vi "Capture Example.vi"() -> ()   [LabVIEW 2020]
uses:
  g_ar_toolkit.image/CreateEmptyImageARGB.vi
  g_ar_toolkit.image/DrawImageToPictureARGB.vi
  g_ar_toolkit.image/CreateEmptyImageARGB.vi/3321fa97-f432-4e1e-8db9-a0df79aed21b.vi
  g_ar_toolkit.image/DrawImageToPictureARGB.vi/8cd07b1b-062e-4fe4-9e87-2eb3dc89fe0e.vi
  g_ar_toolkit.image/ARGBColourToU32.vi
  <vilib>/Utility/error.llb/Error Cluster From Error Code.vi
  g_ar_toolkit.capture/CameraStream/CameraStream.lvclass
  g_ar_toolkit.capture/CameraManager/CameraManager.lvclass
  g_ar_toolkit.image/g_ar_toolkit.image.lvlib
panel:
  in  "Start/Stop":bool
  in  "Format":string(combo)
  in  "Source":string(combo)
  in  "Enumerate":bool
  in  "Erase":bool
  in  "Picture Zoom":dbl=1.0 min=0.0001 max=10.0 step=0.1
  out "2D Picture":picture
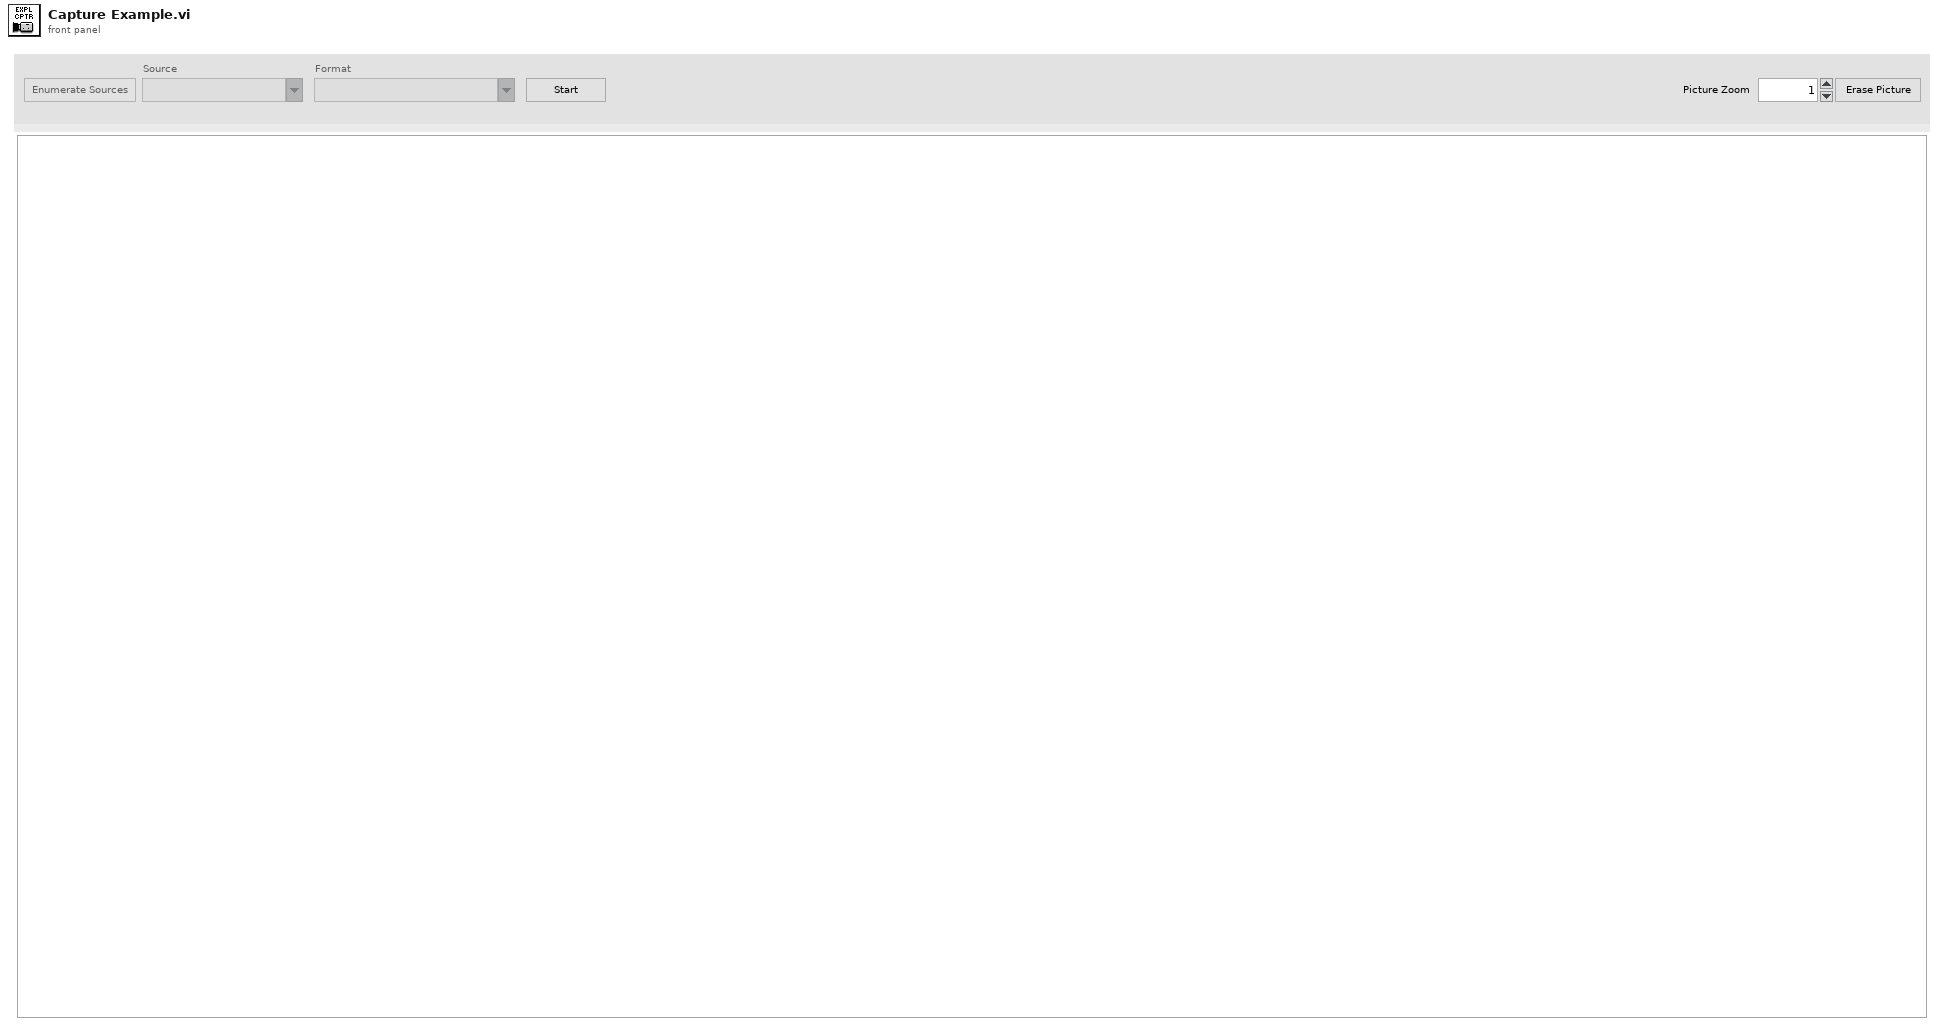
[diagram p1: front panel]
types:
  T1 = enum8{"Enabled", "Disabled", "Disabled and Grayed Out"}
  T2 = typedef "g_ar_toolkit.capture.lvlib/CameraManager.lvclass/Device Enumeration.ctl" = cluster{"Name":string, "Streams":set{cluster{"Parameters":T3, "Pixel-Format":u32, "Pixel-Format Name":string}}}
  T3 = typedef "g_ar_toolkit.capture.lvlib/CameraManager.lvclass/Stream Parameters.ctl" = cluster{"Width":u16, "Height":u16, "FPS":u8}
  T4 = set{cluster{"Parameters":T3, "Pixel-Format":u32, "Pixel-Format Name":string}}
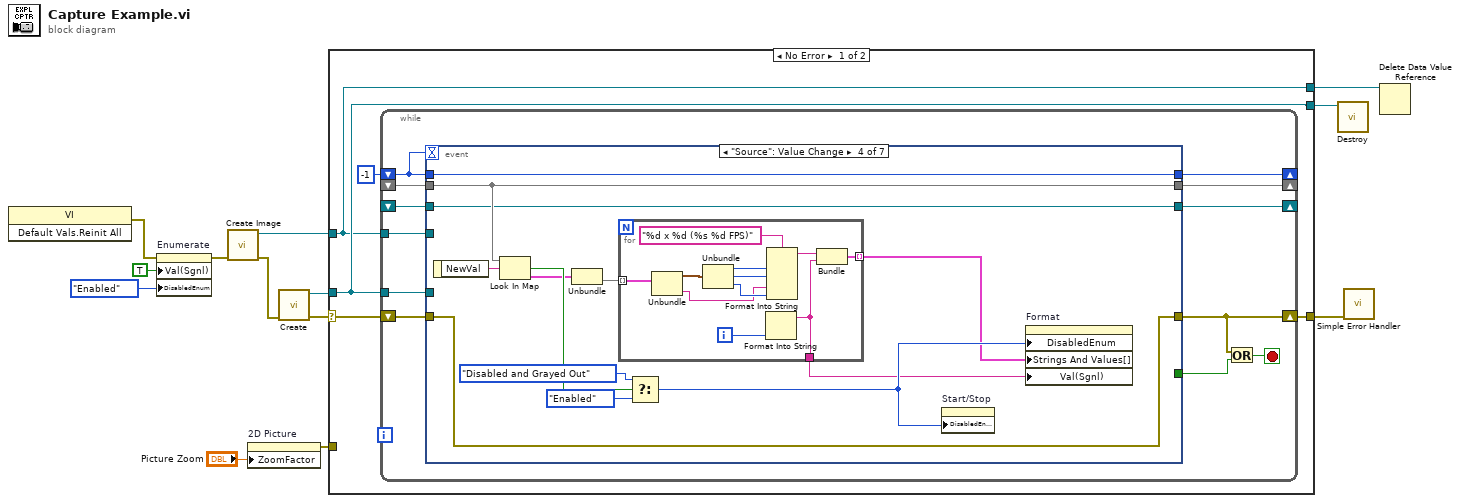
[diagram p0: block diagram]
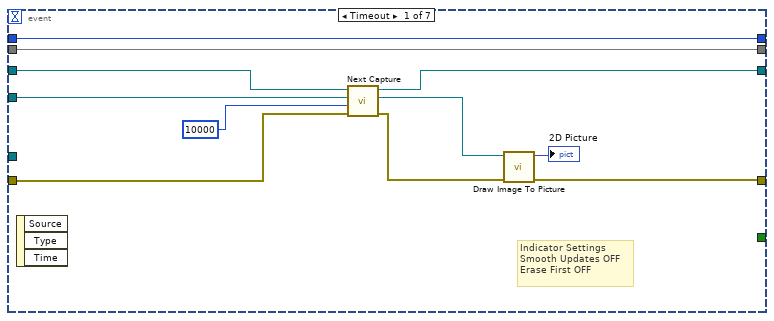
[diagram p2: hidden frame]
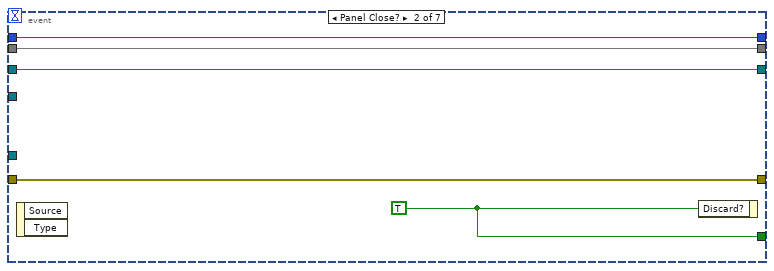
[diagram p3: hidden frame]
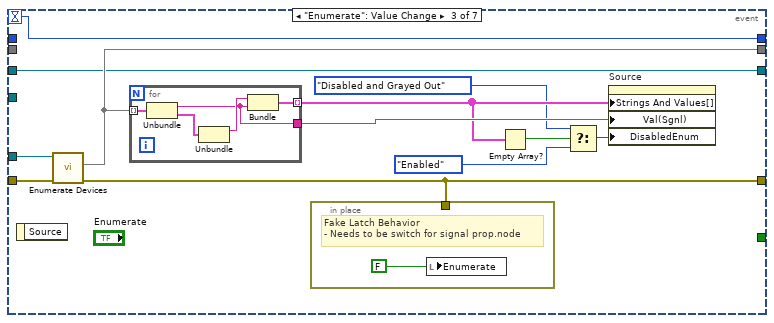
[diagram p4: hidden frame]
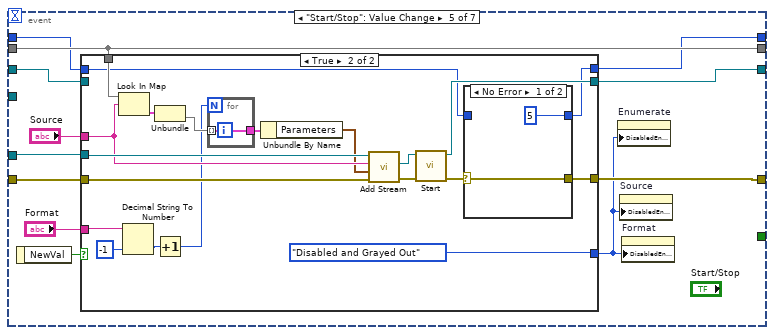
[diagram p5: hidden frame]
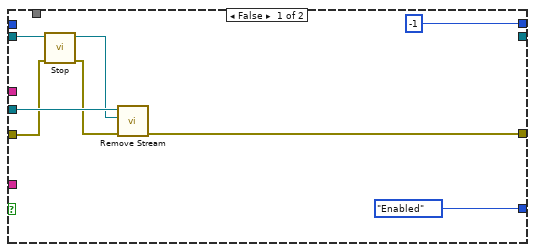
[diagram p6: hidden frame]
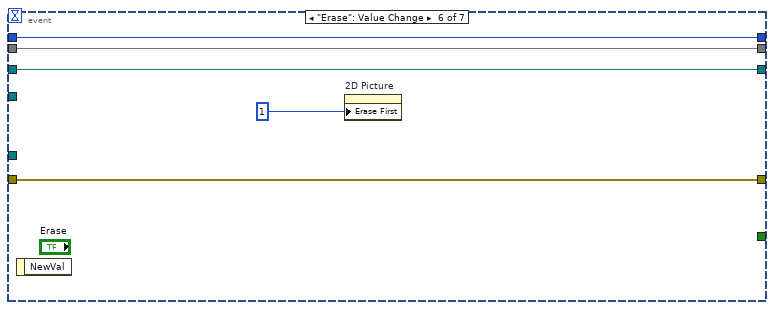
[diagram p8: hidden frame]
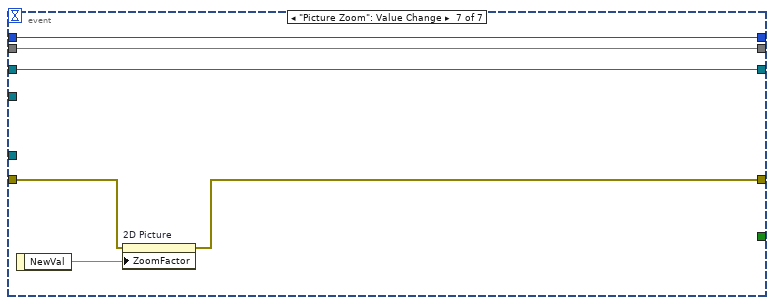
[diagram p9: hidden frame]
diagram:
  n1 = invoke class="VI" method="Default Vals.Reinit All"() -> (error out=w5:errorcluster)  [unwired: 3 in, 2 out]
  n2 = property on="Enumerate" class="Bool (strict)"(error in=w5, "Val(Sgnl)"=TRUE ("Value (Signaling)"), "DisabledEnum"=T1."Enabled" ("Disabled")) -> (error out=w1:errorcluster)  [unwired: 1 in, 1 out]
  n3 = call-poly "Create Image.vi"("error in (no error)"=w1) -> ("error out"=w4:errorcluster, "New ARGB Image"=w10:refnum<data-value>)  [unwired: 9 in]
  n4 = property on="2D Picture" class="Pict"("ZoomFactor"="Picture Zoom") -> (error out=w9:errorcluster)  [unwired: 2 in, 1 out]
  n5 = call "Create.vi"("error in (no error)"=w4) -> ("error out"=w13:errorcluster, "CameraManager"=w2:refnum<data-value>)  [unwired: 9 in]
  n6 = case shown="No Error" w13 {
    selector: w13 -> [w18 w145]
    tunnel: w2 -> [w17 w147]
    tunnel: [w17 w147] -> w12
    tunnel: w10 -> [w15 w146]
    tunnel: w9 -> [_ _]
    tunnel: [w15 w146] -> w7
    tunnel: [w14 w145] -> w6
    frame No Error {
      n7 = while {
        tunnel: w17 -> [w30]
        shift-right: [w28] -> _
        shift-left: _ -> [w27]
        shift-right: [w26] -> w14
        shift-left: w18 -> [w29]
        shift-right: [w23] -> _
        shift-left: -1 -> [w22]
        shift-right: [w21] -> _
        shift-left: _ -> [w20]
        tunnel: w15 -> [w19]
        stop <- w25 stop-if-true
        n8 = event shown="[3] \"Source\": Value Change" {
          selector: _ -> [_ _ _ _ _ _ _]
          dyn-events: _ -> [_ _ _ _ _ _ _]
          timeout: w22 -> [_ _ w53 _ _ _ _]
          tunnel: w30 -> [_ _ w58 _ w96 _ _]
          tunnel: w29 -> [w33 w45 w57 w65 w97 w135 w141]
          tunnel: [w41 w44 w56 w77 w95 w138 w139] -> w28
          tunnel: w27 -> [w41 w44 _ w77 w95 w138 w139]
          tunnel: [w32 w45 w54 w65 w94 w135 w140] -> w26
          tunnel: [_ w46 _ _ _ _ _] -> w24
          tunnel: [w40 w43 w53 w67 w91 w137 w144] -> w23
          tunnel: w22 -> [w40 w43 _ w67 w92 w137 w144]
          tunnel: [w38 w42 w52 w66 w93 w136 w143] -> w21
          tunnel: w20 -> [w39 w42 w52 w66 w90 w136 w143]
          tunnel: w19 -> [w37 _ _ _ _ _ _]
          event Timeout {
            # "Indicator Settings\nSmooth Updates OFF\nErase First OFF"
            n9 = event-data() -> ()  [unwired: 1 in, 3 out]
            n10 = call "Next Capture.vi"("error in (no error)"=w33, "timeout (ms)"=u16 10000, "ARGB Image Destination"=w37, "Stream"=w39) -> ("error out"=w34:errorcluster, "ARGB Image (duplicate)"=w35:refnum<data-value>, "Stream (duplicate)"=w38:refnum<data-value>)  [unwired: 5 in]
            n11 = call-poly "Draw Image To Picture.vi"("error in (no error)"=w34, "ARGB Image Source"=w35) -> ("error out"=w32:errorcluster, "Picture"=→"2D Picture":picture)  [unwired: 8 in]
          }
          event Panel Close? {
            w46 = TRUE ("Discard?")
            n12 = event-data() -> ()  [unwired: 1 in, 2 out]
            n13 = event-data("Discard?"=w46) -> ()  [unwired: 1 in, 1 out]
          }
          event "Enumerate": Value Change {
            n14 = event-data() -> ()  [unwired: 1 in, 1 out]
            n15 = call "Enumerate Devices.vi"("error in (no error)"=w57, "CameraManager"=w58) -> ("error out"=w54:errorcluster, "Devices"=w56:map{string, T2})  [unwired: 7 in, 1 out]
            n16 = for {
              tunnel: w56 -> [w64] mode=indexing
              tunnel: [w61] -> w50 mode=indexing
              tunnel: [w60] -> w55
              n17 = Unbundle(w64) -> ("id"=w60:string, "Device Enumeration"=w63:T2)
              n18 = Unbundle(w63) -> ("Name"=w62:string)  [unwired: 1 out]
              n19 = Bundle("Name"=w62, "id"=w60) -> (w61:cluster{"Name":string, "id":string})  [unwired: 1 in]
            }
            n20 = in-place {
              in-place-border: w54 -> [_]
              # "Fake Latch Behavior\n- Needs to be switch for signal prop.node"
              n21 = local write "Enumerate"(FALSE ("Re-Enumerate Sources")) -> ()
            }
            n22 = Empty Array?(array=w50) -> (empty?=w51:bool)
            n23 = Select(t=T1."Disabled and Grayed Out", s=w51, f=T1."Enabled" ("Disabled")) -> (s? t:f=w47:T1)
            n24 = property on="Source" class="CmbBox"("Strings And Values[]"=w50, "Val(Sgnl)"=w55, "DisabledEnum"=w47) -> ()  [unwired: 2 in, 2 out]
          }
          event "Source": Value Change {
            n25 = event-data() -> ("NewVal"=w76:string)  [unwired: 1 in]
            n26 = Look In Map(map=w77, key=w76) -> (key not found?=w75:bool, value=w72:T2)  [unwired: 1 in]
            n27 = Unbundle(w72) -> ("Streams"=w71:T4)  [unwired: 1 out]
            n28 = for {
              tunnel: w71 -> [w83] mode=indexing
              tunnel: [w86] -> w69 mode=indexing
              tunnel: [w85] -> w68
              i -> [w88]
              n29 = Unbundle(w83) -> ("Parameters"=w82:T3, "Pixel-Format Name"=w78:string)  [unwired: 1 out]
              n30 = Unbundle(w82) -> ("Width"=w81:u16, "Height"=w80:u16, "FPS"=w79:u8)
              n31 = Format Into String(w88) -> (resulting string=w85:string)  [unwired: 3 in, 1 out]
              n32 = Format Into String(format string="%d x %d (%s %d FPS)", w81, w80, w78, w79) -> (resulting string=w87:string)  [unwired: 2 in, 1 out]
              n33 = Bundle(w87, w85) -> (w86:cluster{string, string})  [unwired: 1 in]
            }
            n34 = Select(t=T1."Disabled and Grayed Out" ("Disabled"), s=w75, f=T1."Enabled") -> (s? t:f=w70:T1)
            n35 = property on="Start/Stop" class="Bool (strict)"("DisabledEnum"=w70) -> ()  [unwired: 2 in, 2 out]
            n36 = property on="Format" class="CmbBox"("DisabledEnum"=w70, "Strings And Values[]"=w69, "Val(Sgnl)"=w68) -> ()  [unwired: 2 in, 2 out]
          }
          event "Start/Stop": Value Change {
            n37 = event-data() -> ("NewVal"=w100:bool)  [unwired: 1 in]
            n38 = case shown="True" w100 {
              tunnel: "Source" -> [_ w124]
              tunnel: "Format" -> [_ w123]
              tunnel: w97 -> [w105 w127]
              tunnel: w96 -> [w107 w128]
              tunnel: w95 -> [_ w126]
              tunnel: [w102 w118] -> w94
              tunnel: [_ w116] -> w93
              tunnel: w92 -> [_ w115]
              tunnel: [-1 w114] -> w91
              tunnel: w90 -> [w108 _]
              tunnel: [T1."Enabled" ("Disabled") T1."Disabled and Grayed Out" ("Disabled")] -> w89
              frame False {
                n39 = call "Stop.vi"("error in (no error)"=w105, "Stream"=w108) -> ("error out"=w104:errorcluster, "Stream (duplicate)"=w106:refnum<data-value>)  [unwired: 8 in]
                n40 = call "Remove Stream.vi"("error in (no error)"=w104, "Stream"=w106, "CameraManager"=w107) -> ("error out"=w102:errorcluster)  [unwired: 7 in, 1 out]
              }
              frame True {
                n41 = Look In Map(map=w126, key=w124) -> (value=w125:T2)  [unwired: 1 in, 1 out]
                n42 = Decimal String To Number(string=w123, default (0L)=-1 ("default (0 I32)")) -> (number=w119:i32)  [unwired: 1 in, 1 out]
                n43 = Unbundle(w125) -> ("Streams"=w122:T4)  [unwired: 1 out]
                n44 = Increment(x=w119) -> (x+1=w120:i32)
                n45 = for {
                  N: w120 -> [_]
                  tunnel: w122 -> [w133] mode=indexing
                  tunnel: [w133] -> w110
                }
                n46 = Unbundle By Name(w110) -> ("Parameters"=w109:T3)
                n47 = call "Add Stream.vi"("error in (no error)"=w127, "Desired Stream Parameters"=w109, "Device ID"=w124, "CameraManager"=w128) -> ("error out"=w112:errorcluster, "Stream"=w113:refnum<data-value>)  [unwired: 5 in, 1 out]
                n48 = call "Start.vi"("error in (no error)"=w112, "Stream"=w113) -> ("error out"=w117:errorcluster, "Stream (duplicate)"=w116:refnum<data-value>)  [unwired: 8 in]
                n49 = case shown="No Error" w117 {
                  selector: w117 -> [w130 w131]
                  tunnel: [w130 w131] -> w118
                  tunnel: w115 -> [_ w132]
                  tunnel: [5 w132] -> w114
                  frame No Error {
                  }
                  frame Error {
                  }
                }
              }
            }
            n50 = property on="Enumerate" class="Bool (strict)"("DisabledEnum"=w89) -> ()  [unwired: 2 in, 2 out]
            n51 = property on="Source" class="CmbBox"("DisabledEnum"=w89) -> ()  [unwired: 2 in, 2 out]
            n52 = property on="Format" class="CmbBox"("DisabledEnum"=w89) -> ()  [unwired: 2 in, 2 out]
          }
          event "Erase": Value Change {
            n53 = event-data() -> ()  [unwired: 1 in, 1 out]
            n54 = property on="2D Picture" class="Pict"("Erase First"=u8 1) -> ()  [unwired: 2 in, 2 out]
          }
          event "Picture Zoom": Value Change {
            n55 = event-data() -> ("NewVal"=w142:dbl)  [unwired: 1 in]
            n56 = property on="2D Picture" class="Pict"(error in=w141, "ZoomFactor"=w142) -> (error out=w140:errorcluster)  [unwired: 1 in, 1 out]
          }
        }
        n57 = Or(x=w26, y=w24) -> (x .or. y?=w25:bool)
      }
    }
    frame Error {
    }
  }
  n58 = call "Destroy.vi"("CameraManager"=w12) -> ()  [unwired: 10 in, 1 out]
  n59 = call <vilib>:"Simple Error Handler.vi"("error in (no error)"=w6) -> ()  [unwired: 4 in, 5 out]
  n60 = Delete Data Value Reference(data value reference=w7) -> ()  [unwired: 1 in, 2 out]
